vi "String array to semicolon.vi"(8 "error in":errorcluster, 11 "String array":string[](array[string])) -> (0 "error out":errorcluster, 3 "Semicolon string":string)   [LabVIEW 2012]
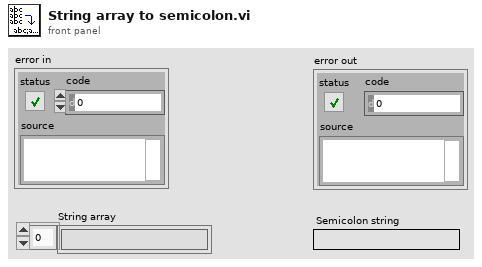
[diagram p1: front panel]
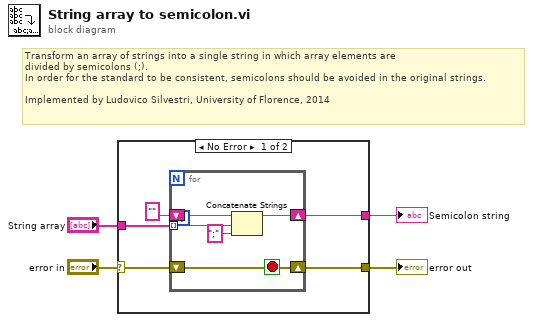
[diagram p0: block diagram]
diagram:
  # "Transform an array of strings into a single string in which array elements are\ndivided by semicolons (;). \nIn order for the standard to be consistent, semicolons should be avoided in the original strings.\n\nImplemented by Ludovico Silvestri, University of Florence, 2014"
  n1 = case shown="No Error" "error in" {
    selector: "error in" -> [w7 w15]
    tunnel: [w6 w15] -> w3
    tunnel: "String array" -> [w9 _]
    tunnel: [w5 _] -> w1
    frame No Error {
      n2 = for {
        tunnel: w9 -> [w13] mode=indexing
        shift-right: [w11] -> w5
        shift-left: "" -> [w14]
        shift-right: [w10] -> w6
        shift-left: w7 -> [w10]
        stop <- w10 stop-if-true
        n3 = Concatenate Strings(w14, w13, ";" ("string")) -> (w11:string)
      }
    }
    frame Error {
    }
  }
  "error out" <- w3
  "Semicolon string" <- w1
